vi "Read.vi"(8 "error in (no error)":errorcluster, 11 "Wifi in":refnum<class "Wifi.lvclass">) -> (0 "error out":errorcluster, 2 "Message":string, 3 "Wifi out":refnum<class "Wifi.lvclass">)   [LabVIEW 2021, in "Wifi.lvclass"]
uses:
  Wifi.lvclass
  Wifi.lvclass/Wifi.ctl
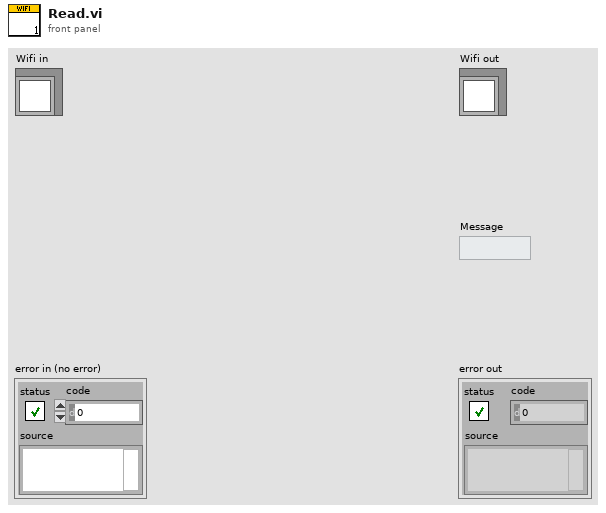
[diagram p1: front panel]
types:
  T1 = enum16{"Standard", "Buffered", "CRLF", "Immediate"}
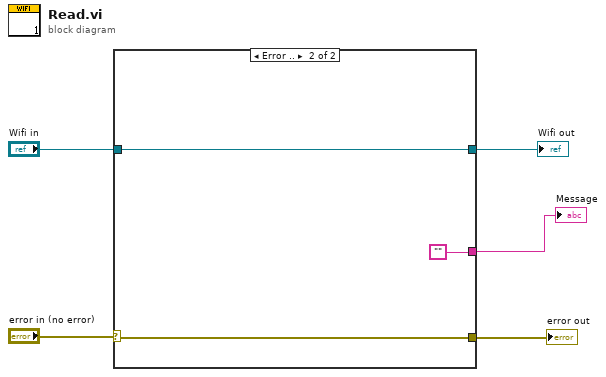
[diagram p0: block diagram]
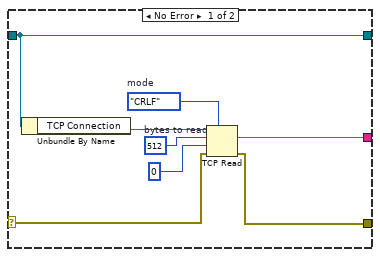
[diagram p2: hidden frame]
diagram:
  n1 = case shown="Error .." "error in (no error)" {
    selector: "error in (no error)" -> [w10 w16]
    tunnel: [w9 w16] -> w4
    tunnel: [w8 ""] -> w3
    tunnel: "Wifi in" -> [w6 w15]
    tunnel: [w6 w15] -> w1
    frame No Error {
      w12 = T1."CRLF"  # mode
      w13 = 512  # bytes to read
      n2 = Unbundle By Name(w6) -> ("TCP Connection"=w7:refnum<k5>)
      n3 = TCP Read(connection ID=w7, bytes to read=w13, error in (no error)=w10, 7:w12, 9:0 ("timeout ms (25000)")) -> (data out=w8:string, error out=w9:errorcluster)  [unwired: 1 out]
    }
    frame Error {
    }
  }
  "error out" <- w4
  "Wifi out" <- w1
  "Message" <- w3
